vi "Read C2.vi"(8 "error in (no error)":errorcluster, 11 "My Custom Type in":refnum<class "My Custom Type.lvclass">) -> (0 "error out":errorcluster, 2 "fieldE":dbl, 3 "My Custom Type out":refnum<class "My Custom Type.lvclass">)   [LabVIEW 2020, in "My Custom Type.lvclass"]
uses:
  My Custom Type.lvclass
  My Custom Type.lvclass/My Custom Type.ctl
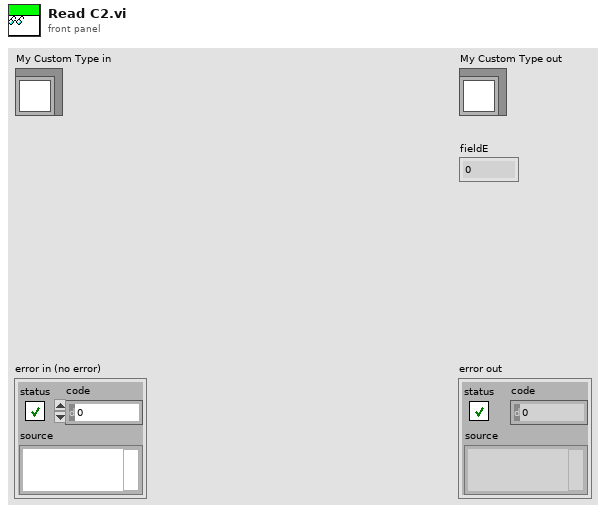
[diagram p1: front panel]
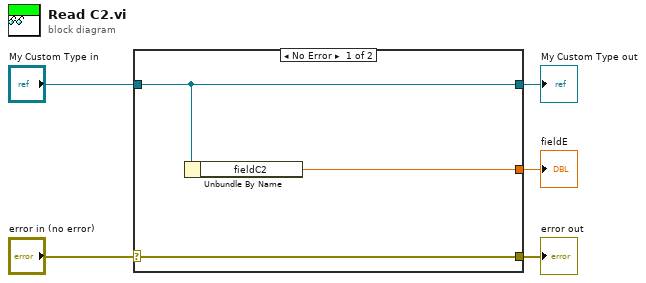
[diagram p0: block diagram]
diagram:
  n1 = case shown="No Error" "error in (no error)" {
    selector: "error in (no error)" -> [w8 w9]
    tunnel: [w8 w9] -> w4
    tunnel: [w7 w10] -> w2
    tunnel: "My Custom Type in" -> [w7 w10]
    tunnel: [w6 _] -> w1
    frame No Error {
      n2 = Unbundle By Name(w7) -> ("fieldC2"=w6:dbl)
    }
    frame Error {
    }
  }
  "error out" <- w4
  "My Custom Type out" <- w2
  "fieldE" <- w1
